vi "Set Strings from Ref.vi"(8 "error in (no error)":errorcluster, 9 "Language Index (0)":i32, 10 "GObj Refnum":refnum<vi>, 11 "WaveformGraph in":refnum<class "WaveformChart.lvclass">) -> (0 "error out":errorcluster, 3 "WaveformGraph out":refnum<class "WaveformChart.lvclass">)   [LabVIEW 2013, in "SET Project Data.lvlib" / "WaveformChart.lvclass"]
uses:
  WaveformChart.lvclass
  GraphChart/GraphChart.lvclass
  GObject/GObject.lvclass
  SET Project Data.lvlib
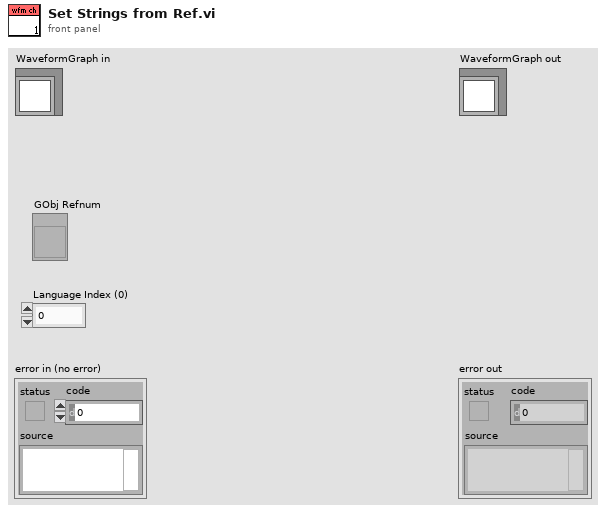
[diagram p1: front panel]
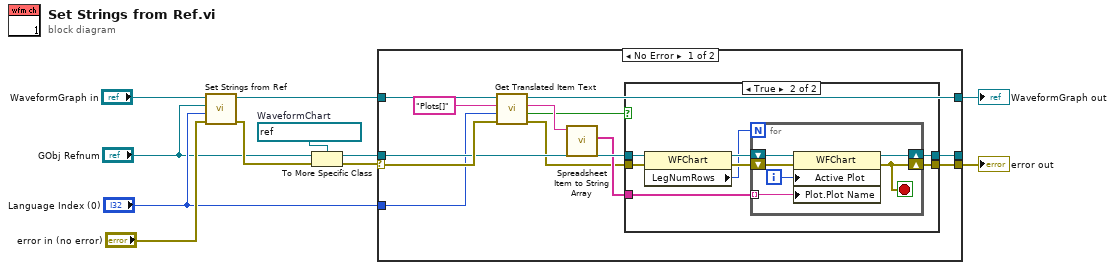
[diagram p0: block diagram]
diagram:
  w7 = refnum<vi> refnum  # WaveformChart
  n1 = call-parent "Set Strings from Ref.vi"("error in (no error)"="error in (no error)", "Language Index (0)"="Language Index (0)", "GObj Refnum"="GObj Refnum", "GraphChart in"="WaveformGraph in") -> ("error out"=w5:errorcluster, "GraphChart out"=w6:refnum<class "WaveformChart.lvclass">)  [unwired: 6 in]
  n2 = To More Specific Class(target class=w7, reference="GObj Refnum", error in=w5) -> (specific class reference=w9:refnum<vi>, error out=w8:errorcluster)
  n3 = case shown="No Error" w8 {
    selector: w8 -> [w20 w41]
    tunnel: w9 -> [w18 w40]
    tunnel: w6 -> [w22 w42]
    tunnel: "Language Index (0)" -> [w15 _]
    tunnel: [w14 w42] -> w2
    tunnel: [w12 w41] -> w1
    tunnel: [w13 w40] -> _
    frame No Error {
      n4 = call "Get Translated Item Text.vi"("error in (no error)"=w20, "LangIndex (0)"=w15, "ItemName"="Plots[]", "GObject in"=w22) -> ("error out"=w16:errorcluster, "Found?"=w19:bool, "Translated Text (ASCII)"=w21:string, "GObject out"=w14:refnum<class "WaveformChart.lvclass">)  [unwired: 4 in]
      n5 = call "Spreadsheet Item to String Array.vi"("Spreadsheet Item (ASCII)"=w21) -> ("Strings [] (ASCII)"=w17:string[])  [unwired: 10 in]
      n6 = case shown="True" w19 {
        tunnel: w18 -> [w24 w30]
        tunnel: w17 -> [_ w33]
        tunnel: w16 -> [w25 w29]
        tunnel: [w25 w32] -> w12
        tunnel: [w24 w31] -> w13
        frame False {
        }
        frame True {
          n7 = property class="WFChart"(reference=w30, error in=w29) -> (reference out=w28:refnum<vi>, error out=w27:errorcluster, "LegNumRows"=w26:u32)
          n8 = for {
            N: w26 -> [_]
            tunnel: w33 -> [w37] mode=indexing
            shift-right: [w36] -> w31
            shift-left: w28 -> [w39]
            shift-right: [w34] -> w32
            shift-left: w27 -> [w35]
            i -> [w38]
            stop <- w34 stop-if-true
            n9 = property class="WFChart"(reference=w39, error in=w35, "Active Plot"=w38, "Plot.Plot Name"=w37) -> (reference out=w36:refnum<vi>, error out=w34:errorcluster)
          }
        }
      }
    }
    frame Error {
    }
  }
  "error out" <- w1
  "WaveformGraph out" <- w2
